vi "Save Data I16.vi"(8 "error in (no error)":errorcluster, 9 "I32 data":i32[][](array[numeric]), 10 "I16 data":i16[][](array[numeric]), 11 "DAQmx Synthesizer in":refnum<class "DAQmx Synthesizer.lvclass">) -> (0 "error out":errorcluster, 3 "DAQmx Synthesizer out":refnum<class "DAQmx Synthesizer.lvclass">)   [LabVIEW 2019, in "DAQmx Synthesizer.lvclass"]
uses:
  DAQmx Synthesizer.lvclass
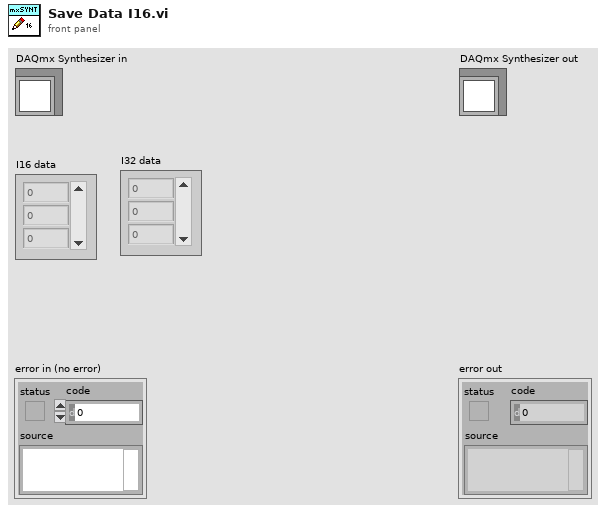
[diagram p1: front panel]
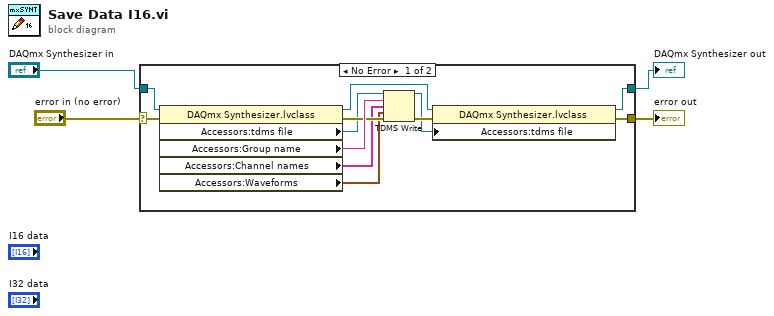
[diagram p0: block diagram]
diagram:
  n1 = case shown="No Error" "error in (no error)" {
    selector: "error in (no error)" -> [w10 w18]
    tunnel: [w9 w18] -> w2
    tunnel: [w7 w17] -> w3
    tunnel: "DAQmx Synthesizer in" -> [w12 w17]
    frame No Error {
      n2 = property class="DAQmx Synthesizer.lvclass"(reference=w12, error in=w10) -> (reference out=w8:refnum<class "DAQmx Synthesizer.lvclass">, error out=w15:errorcluster, "Accessors:tdms file"=w13:refnum<k34>, "Accessors:Group name"=w16:string, "Accessors:Channel names"=w14:string[], "Accessors:Waveforms"=w5:waveform(dbl)[])
      n3 = TDMS Write(0:w13, 5:w16, 7:w14, 9:w5, 11:w15) -> (4:w6:refnum<k34>, 15:w11:errorcluster)  [unwired: 1 in, 2 out]
      n4 = property class="DAQmx Synthesizer.lvclass"(reference=w8, error in=w11, "Accessors:tdms file"=w6) -> (reference out=w7:refnum<class "DAQmx Synthesizer.lvclass">, error out=w9:errorcluster)
    }
    frame Error {
    }
  }
  "error out" <- w2
  "DAQmx Synthesizer out" <- w3
